vi "Initialize control (SubVI).vi"(8 "error in (no error)":errorcluster) -> (0 "error out":errorcluster, 3 "Control taken?":bool)   [LabVIEW 2016]
uses:
  <vilib>/Utility/sysdir.llb/System Directory Type.ctl
  <vilib>/Utility/config.llb/Read Key (String).vi
  <vilib>/Utility/config.llb/NI_LVConfig.lvlib
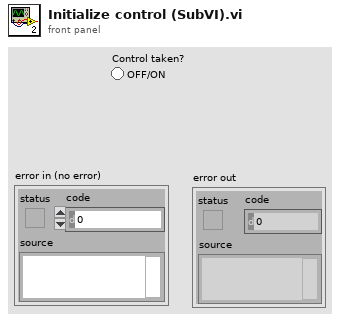
[diagram p1: front panel]
types:
  T1 = typedef "System Directory Type.ctl" = i32
  T2 = typedef "NI_LVConfig.lvlib/Config Data RefNum.ctl" = refnum<k1>
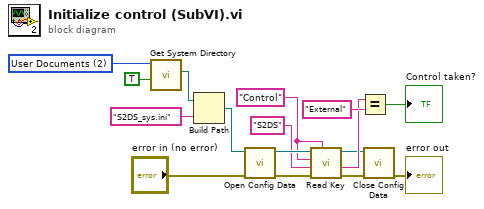
[diagram p0: block diagram]
diagram:
  w7 = "Control" ("section")
  w10 = T1 2 items=["User Home"=0, "User Desktop"=1, "User Documents"=2, "User Application Data"=3, "User Preferences"=4, "User Temporary"=5, "Public Documents"=6, "Public Application Data"=7, "Public Preferences"=8, "Public Cache"=13, "System Core Libraries"=9, "System Installed Libraries"=10, "Application Files"=11, "Boot Volume Root"=12] ("system directory type")
  n1 = call <vilib>:"Get System Directory.vi"("create directory if not found? (F)"=TRUE, "system directory type"=w10) -> ("system directory"=w12:path)  [unwired: 9 in]
  n2 = Build Path(base path=w12, name or relative path="S2DS_sys.ini") -> (appended path=w9:path)
  n3 = call <vilib>:"Open Config Data.vi"("error in (no error)"="error in (no error)", "configuration file path"=w9) -> ("error out"=w3:errorcluster, "refnum"=w8:T2)  [unwired: 7 in, 1 out]
  n4 = call-poly <vilib>:"Read Key.vi"("section"=w7, "error in (no error)"=w3, "default value"="S2DS", "key"=w7, "refnum"=w8) -> ("error out"=w1:errorcluster, "value"=w4:string, "refnum out"=w2:T2)  [unwired: 3 in, 1 out]
  n5 = Equal?(x=w4, y="External") -> (x = y?=→"Control taken?":bool)
  n6 = call <vilib>:"Close Config Data.vi"("error in (no error)"=w1, "refnum"=w2) -> ("error out"=→"error out":errorcluster)  [unwired: 8 in, 1 out]
